vi "Read hFPGA.vi"(8 "error in (no error)":errorcluster, 11 "nPAS in":refnum<class "nPAS.lvclass">) -> (0 "error out":errorcluster, 2 "Session Handle":T1, 3 "nPAS out":refnum<class "nPAS.lvclass">)   [LabVIEW 2016, in "gPAS Library.lvlib" / "nPAS.lvclass"]
uses:
  nPAS.lvclass
  <vilib>/MSR Consulting, LLC/General Reuse/Typedefs/Session Handle.ctl
  <vilib>/MSR Consulting, LLC/General Reuse/Session APIs/_Session Fwk/Session - Root.lvclass
  nPAS.lvclass/nPAS.ctl
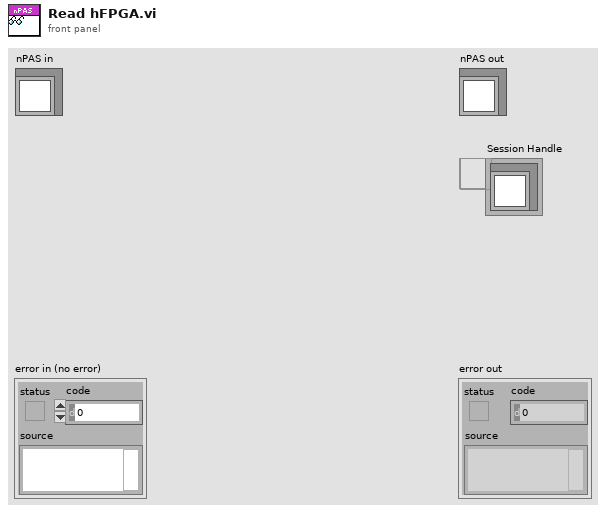
[diagram p1: front panel]
types:
  T1 = typedef "Session - Root.lvclass/Session Handle.ctl" = refnum<data-value>
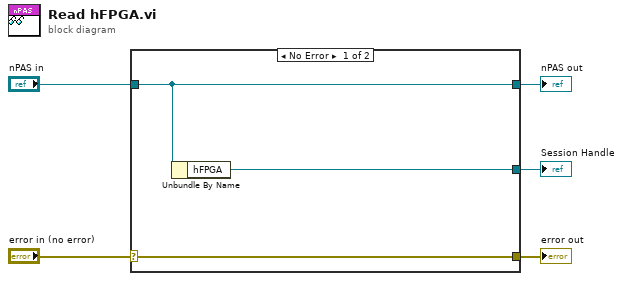
[diagram p0: block diagram]
diagram:
  n1 = case shown="No Error" "error in (no error)" {
    selector: "error in (no error)" -> [w8 w9]
    tunnel: [w8 w9] -> w4
    tunnel: [w7 w10] -> w2
    tunnel: "nPAS in" -> [w7 w10]
    tunnel: [w6 _] -> w1
    frame No Error {
      n2 = Unbundle By Name(w7) -> ("hFPGA"=w6:T1)
    }
    frame Error {
    }
  }
  "error out" <- w4
  "nPAS out" <- w2
  "Session Handle" <- w1
